vi "goqr.vi"(8 "error in (no error)":errorcluster) -> (0 "error out":errorcluster)   [LabVIEW 2019]
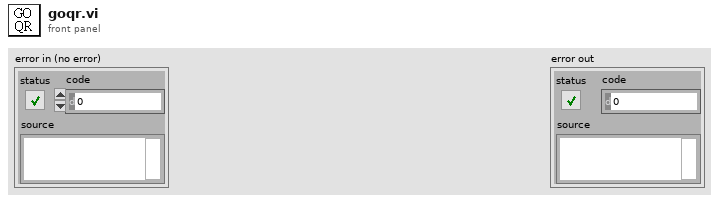
[diagram p1: front panel]
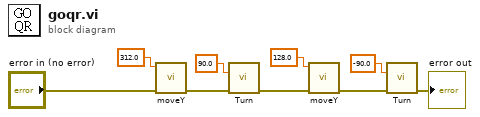
[diagram p0: block diagram]
diagram:
  n1 = call "moveY.vi"("error in (no error)"="error in (no error)", "Y"=312.0) -> ("error out"=w8:errorcluster)  [unwired: 9 in]
  n2 = call "Turn.vi"("¨¤«×"=90.0, "error in (no error)"=w8) -> ("error out"=w5:errorcluster)  [unwired: 13 in]
  n3 = call "moveY.vi"("error in (no error)"=w5, "Y"=128.0) -> ("error out"=w3:errorcluster)  [unwired: 9 in]
  n4 = call "Turn.vi"("¨¤«×"=-90.0, "error in (no error)"=w3) -> ("error out"=→"error out":errorcluster)  [unwired: 13 in]
